vi "Convert RPM to FPS.vi"(5 "RevMotor/RevWheel":dbl=6.67 format="%#_13g", 7 "Wheel Diameter (in)":dbl=4.0 format="%#_13g", 11 "Motor Speed (RPM)":dbl) -> (3 "Translation Speed (FPS)":dbl)   [LabVIEW 2023, in "TShirtWork-SwerveDrive_ACT_ts.lvlib"]
uses:
  TShirtWork-SwerveDrive_ACT_ts.lvlib
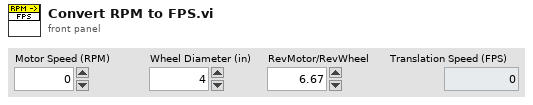
[diagram p1: front panel]
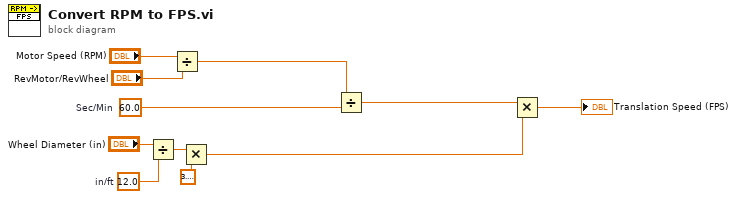
[diagram p0: block diagram]
diagram:
  w3 = 60.0  # Sec/Min
  w10 = 12.0  # in/ft
  n1 = Divide(x="Wheel Diameter (in)", y=w10) -> (x/y=w8:dbl)
  n2 = Divide(x="Motor Speed (RPM)", y="RevMotor/RevWheel") -> (x/y=w5:dbl)
  n3 = Multiply(x=w8, y=3.141592653589793) -> (x*y=w4:dbl)
  n4 = Divide(x=w5, y=w3) -> (x/y=w2:dbl)
  n5 = Multiply(x=w2, y=w4) -> (x*y=→"Translation Speed (FPS)":dbl)
